vi "TORC-TapeMeasureAutonomousManual.vi"(10 "Target Speed":dbl) -> ()   [LabVIEW 2014]
doc: "One of the VIs created by TORC 2137 to control the tape measure. Place this within your code's Autonomous Independent.vi.\n\nThis VI will simply set the speed of the tape measure. Handling of timing should occur outside of the loop.\n\nThere is only one required input; this is the target speed for the tape measure. This value is a motor speed from -1 to 1."
uses:
  TORC-TapeMeasureGlobal.vi
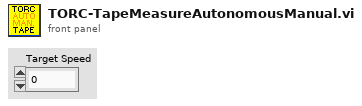
[diagram p1: front panel]
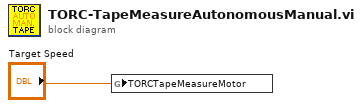
[diagram p0: block diagram]
diagram:
  n1 = global write "TORC-TapeMeasureGlobal.vi" "TORCTapeMeasureMotor"("Target Speed") -> ()
